vi "C400_module.vi"() -> ()   [LabVIEW 2018]
uses:
  data/resilio/Dropbox/rnd/LabView/2p_scanners/notifiers/EventNames.ctl
  data/resilio/Dropbox/rnd/LabView/2p_scanners/notifiers/notifierMessages.ctl
panel:
  in  "autoconnect":bool=TRUE
  out "Ch1 Position Units":string
  out "Ch1Range":i32
  in  "Read Sensor":bool
  out "Ch1 Sensor Value":dbl format="%.3f"
  out "Serial Numbers":string[](array[string])
  out "FT_Status":u64(ring) items=["FT_OK", "FT_INVALID_HANDLE", "FT_DEVICE_NOT_FOUND", "FT_DEVICE_NOT_OPENED", "FT_IO_ERROR", "FT_INSUFFICIENT_RESOURCES", "FT_INVALID_PARAMETER", "FT_INVALID_BAUD_RATE", "FT_DEVICE_NOT_OPENED_FOR_ERASE", "FT_DEVICE_NOT_OPENED_FOR_WRITE", "FT_FAILED_TO_WRITE_DEVICE", "FT_EEPROM_READ_FAILED", "FT_EEPROM_WRITE_FAILED", "FT_EEPROM_ERASE_FAILED", "FT_EEPROM_NOT_PRESENT", "FT_EEPROM_NOT_PROGRAMMED", "FT_INVALID_ARGS", "FT_NOT_SUPPORTED", "FT_OTHER_ERROR"]
  in  "Ch1 Position Cmd":dbl format="%.3f"
  in  "Connect":bool
  in  "Stop VI":bool caption="Stop Button"
  in  "Listbox":i32(listbox)=-1
  in  "Handle":u64
  # "FT_Status displays the error type if an\nFTDI USB function did not execute properly."
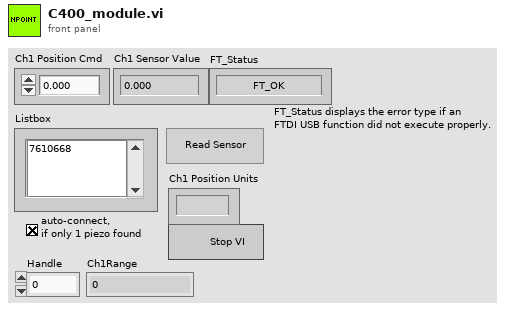
[diagram p1: front panel]
types:
  T1 = typedef "notifierMessages.ctl" = cluster{"data":variant, "source":string, "time tick":u32}
  T2 = typedef "EventNames.ctl" = enum16{"None", "rig shutter", "expStarted", "frameAcq", "stim", "zStage", "DAQ/galvo", "piezo", "liqLens", "expEnded"}
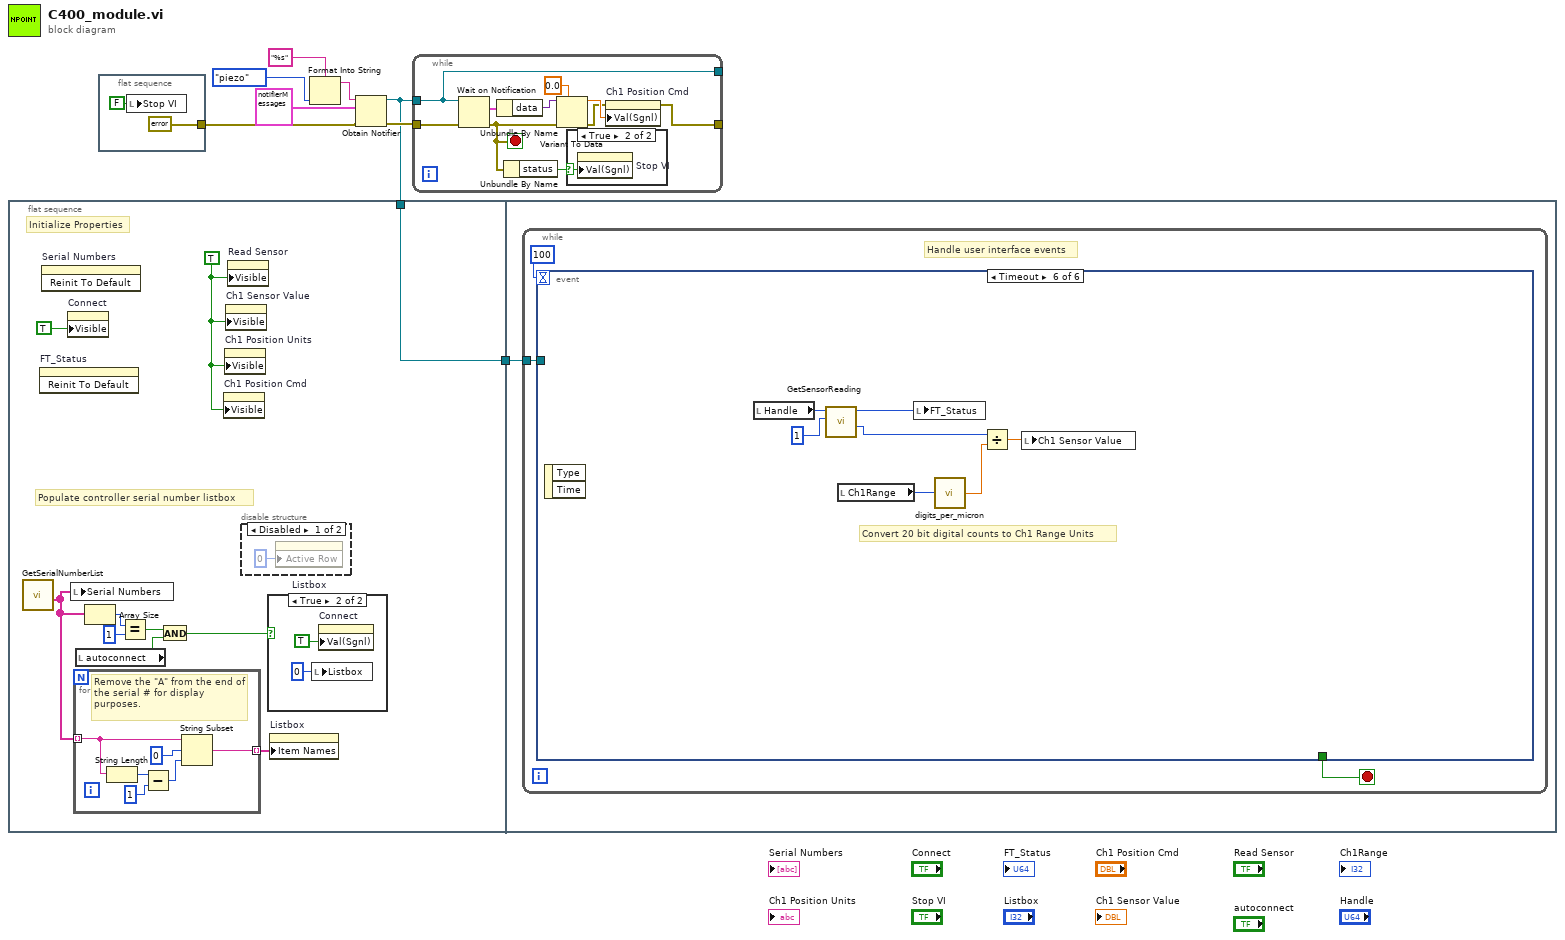
[diagram p0: block diagram]
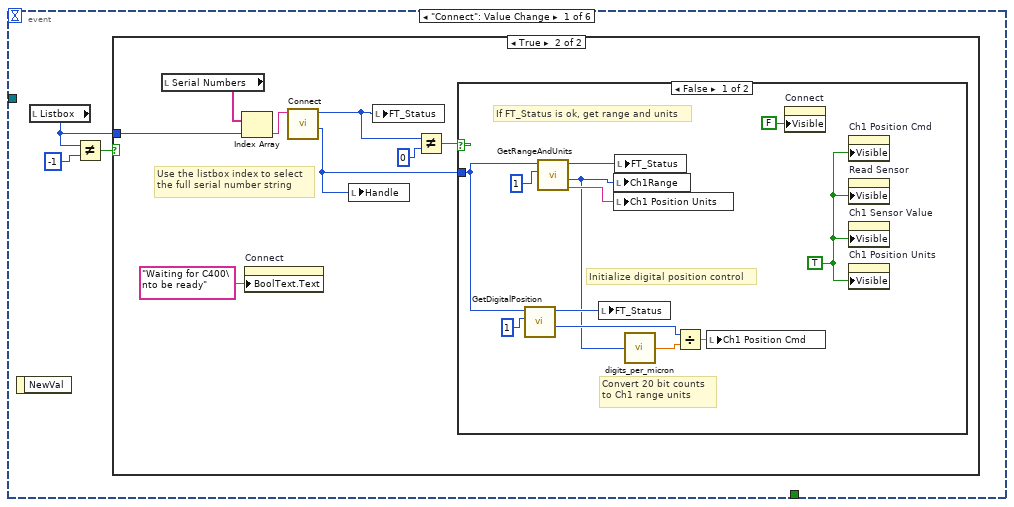
[diagram p5: hidden frame]
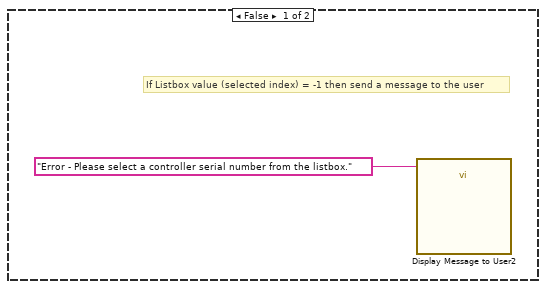
[diagram p6: hidden frame]
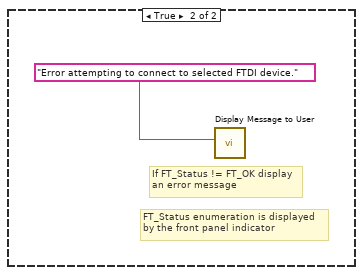
[diagram p7: hidden frame]
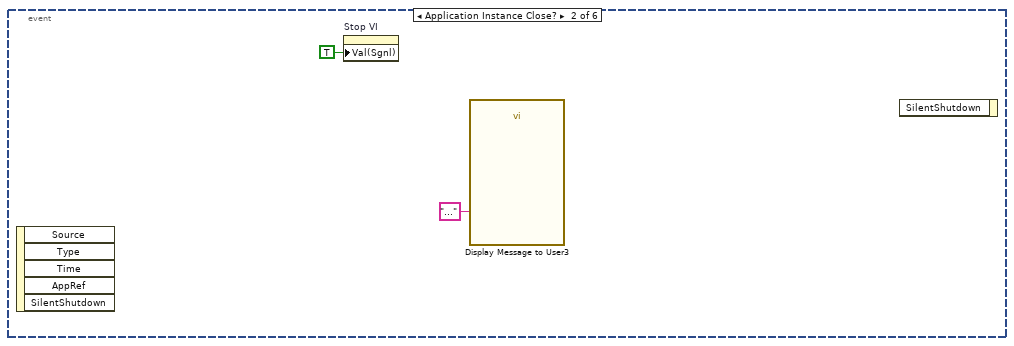
[diagram p8: hidden frame]
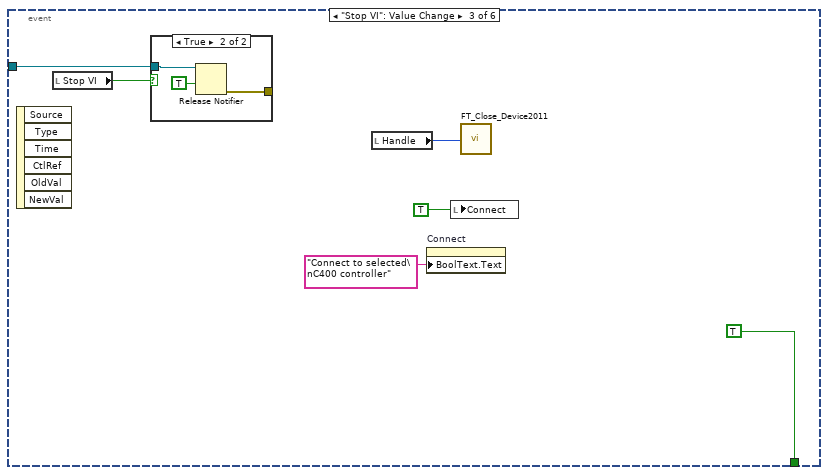
[diagram p9: hidden frame]
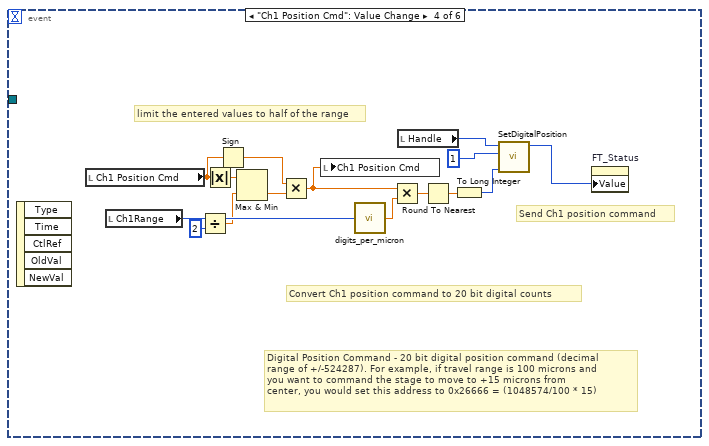
[diagram p11: hidden frame]
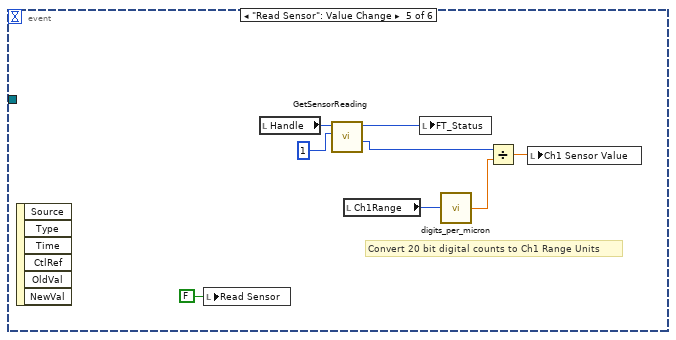
[diagram p12: hidden frame]
diagram:
  n1 = flat-sequence {
    tunnel: w2 -> [w9]
    tunnel: [w9] -> w1
    tunnel: w1 -> [w28]
    frame #0 {
      w16 = TRUE ("Visible")
      # "Initialize Properties"
      # "Populate controller serial number listbox"
      n2 = call "GetSerialNumberList.vi"() -> ("C400 Serial Number Array"=w10:string[])  [unwired: 11 in]
      n3 = invoke on="FT_Status" class="Ring (strict)" method="Reinit To Default"() -> ()  [unwired: 3 in, 3 out]
      n4 = invoke on="Serial Numbers" class="Arr (strict)" method="Reinit To Default"() -> ()  [unwired: 3 in, 3 out]
      n5 = property on="Connect" class="Bool (strict)"("Visible"=TRUE) -> ()  [unwired: 2 in, 2 out]
      n6 = local write "Serial Numbers"(w10) -> ()
      n7 = for {
        tunnel: [w23] -> w18 mode=indexing
        tunnel: w10 -> [w22] mode=indexing
        # "Remove the \"A\" from the end of the serial # for display purposes."
        n8 = String Length(string=w22) -> (length=w26:i32)
        n9 = Subtract(x=w26, y=1) -> (x-y=w24:i32)
        n10 = String Subset(string=w22, offset (0)=0, length (rest)=w24) -> (substring=w23:string)
      }
      n11 = local read "autoconnect"() -> (w12:bool)
      n12 = Array Size(array=w10) -> (size(s)=w14:i32)
      n13 = Equal?(x=w14, y=1) -> (x = y?=w11:bool)
      n14 = And(x=w11, y=w12) -> (x .and. y?=w15:bool)
      n15 = property on="Ch1 Position Cmd" class="DigNum (strict)"("Visible"=w16) -> ()  [unwired: 2 in, 2 out]
      n16 = property on="Ch1 Position Units" class="Str"("Visible"=w16) -> ()  [unwired: 2 in, 2 out]
      n17 = property on="Ch1 Sensor Value" class="DigNum (strict)"("Visible"=w16) -> ()  [unwired: 2 in, 2 out]
      n18 = property on="Read Sensor" class="Bool (strict)"("Visible"=w16) -> ()  [unwired: 2 in, 2 out]
      n19 = disable-structure shown="Disabled" {
        frame Disabled {
          n20 = property on="Listbox" class="LstBox (strict)"("Active Row"=0 ("Active Row:Active Row Number")) -> ()  [unwired: 2 in, 2 out]
        }
        frame Enabled {
        }
      }
      n21 = case shown="True" w15 {
        frame False {
        }
        frame True {
          n22 = local write "Listbox"(0 ("Listbox")) -> ()
          n23 = property on="Connect" class="Bool (strict)"("Val(Sgnl)"=TRUE ("Value (Signaling)")) -> ()  [unwired: 2 in, 2 out]
        }
      }
      n24 = property on="Listbox" class="LstBox (strict)"("Item Names"=w18) -> ()  [unwired: 2 in, 2 out]
    }
    frame #1 {
      n25 = while {
        tunnel: w28 -> [w29]
        stop <- w31 stop-if-true
        # "Handle user interface events"
        n26 = event shown="[5] Timeout" {
          selector: _ -> [_ _ _ _ _ _]
          dyn-events: _ -> [_ _ _ _ _ _]
          timeout: 100 -> [_ _ _ _ _ _]
          tunnel: [_ _ TRUE _ _ _] -> w31
          tunnel: w29 -> [_ _ w59 _ _ _]
          event "Connect": Value Change {
            n27 = event-data() -> ()  [unwired: 1 in, 1 out]
            n28 = local read "Listbox"() -> (w32:i32)
            n29 = Not Equal?(x=w32, y=-1) -> (x != y?=w34:bool)
            n30 = case shown="True" w34 {
              tunnel: w32 -> [_ w43]
              frame False {
                # "If Listbox value (selected index) = -1 then send a message to the user"
                n31 = call "Display Message to User2"("Message"="Error - Please select a controller serial number from the listbox.") -> ()  [unwired: 9 in, 2 out]
              }
              frame True {
                # "Use the listbox index to select\nthe full serial number string"
                n32 = local read "Serial Numbers"() -> (w38:string[])
                n33 = Index Array(array=w38, index=w43) -> (element=w39:string)
                n34 = property on="Connect" class="Bool (strict)"("BoolText.Text"="Waiting for C400\nto be ready" ("Boolean Text.Text")) -> ()  [unwired: 2 in, 2 out]
                n35 = call "Connect.vi"("Device Serial Number"=w39) -> ("Handle"=w42:u64, "FT_Status"=w37:u64)  [unwired: 9 in]
                n36 = local write "Handle"(w42) -> ()
                n37 = local write "FT_Status"(w37) -> ()
                n38 = Not Equal?(x=w37, y=u64 0) -> (x != y?=w40:bool)
                n39 = case shown="False" w40 {
                  tunnel: w42 -> [w49 _]
                  frame False {
                    w46 = TRUE ("Visible")
                    # "Convert 20 bit counts\nto Ch1 range units"
                    # "Initialize digital position control"
                    # "If FT_Status is ok, get range and units"
                    n40 = call "GetDigitalPosition.vi"("Handle"=w49, "Controller Channel"=i64 1) -> ("FT_Status"=w47:u64, "Position"=w53:i64)  [unwired: 7 in]
                    n41 = call "GetRangeAndUnits.vi"("Handle"=w49, "Controller Channel"=i64 1) -> ("FT_Status"=w51:u64, "Range"=w44:i32, "Range Units"=w50:string)  [unwired: 6 in]
                    n42 = local write "FT_Status"(w47) -> ()
                    n43 = local write "Ch1Range"(w44) -> ()
                    n44 = local write "Ch1 Position Units"(w50) -> ()
                    n45 = local write "FT_Status"(w51) -> ()
                    n46 = call "digits_per_micron.vi"("Ch1Range"=w44) -> ("digital_per_micron"=w45:dbl)
                    n47 = Divide(x=w53, y=w45) -> (x/y=w48:dbl)
                    n48 = local write "Ch1 Position Cmd"(w48) -> ()
                    n49 = property on="Connect" class="Bool (strict)"("Visible"=FALSE) -> ()  [unwired: 2 in, 2 out]
                    n50 = property on="Ch1 Position Cmd" class="DigNum (strict)"("Visible"=w46) -> ()  [unwired: 2 in, 2 out]
                    n51 = property on="Read Sensor" class="Bool (strict)"("Visible"=w46) -> ()  [unwired: 2 in, 2 out]
                    n52 = property on="Ch1 Sensor Value" class="DigNum (strict)"("Visible"=w46) -> ()  [unwired: 2 in, 2 out]
                    n53 = property on="Ch1 Position Units" class="Str"("Visible"=w46) -> ()  [unwired: 2 in, 2 out]
                  }
                  frame True {
                    # "FT_Status enumeration is displayed\nby the front panel indicator"
                    # "If FT_Status != FT_OK display\nan error message"
                    n54 = call "Display Message to User"("Message"="Error attempting to connect to selected FTDI device.") -> ()  [unwired: 9 in, 2 out]
                  }
                }
              }
            }
          }
          event Application Instance Close? {
            n55 = event-data() -> ()  [unwired: 1 in, 5 out]
            n56 = property on="Stop VI" class="Bool (strict)"("Val(Sgnl)"=TRUE ("Value (Signaling)")) -> ()  [unwired: 2 in, 2 out]
            n57 = call "Display Message to User3"("Message"="...") -> ()  [unwired: 9 in, 2 out]
            n58 = event-data() -> ()  [unwired: 2 in, 1 out]
          }
          event "Stop VI": Value Change {
            n59 = event-data() -> ()  [unwired: 1 in, 6 out]
            n60 = local read "Stop VI"() -> (w60:bool)
            n61 = case shown="True" w60 {
              tunnel: [_ w66] -> _
              tunnel: w59 -> [_ w65]
              frame False {
              }
              frame True {
                n62 = Release Notifier(notifier=w65, force destroy? (F)=TRUE) -> (error out=w66:errorcluster)  [unwired: 1 in, 2 out]
              }
            }
            n63 = local read "Handle"() -> (w62:u64)
            n64 = property on="Connect" class="Bool (strict)"("BoolText.Text"="Connect to selected\nC400 controller" ("Boolean Text.Text")) -> ()  [unwired: 2 in, 2 out]
            n65 = local write "Connect"(TRUE ("Visible")) -> ()
            n66 = call "FT_Close_Device2011.vi"("Handle"=w62) -> ()  [unwired: 1 out]
          }
          event "Ch1 Position Cmd": Value Change {
            # "limit the entered values to half of the range"
            # "Digital Position Command - 20 bit digital position command (decimal\nrange of +/-524287). For example, if travel range is 100 microns and\nyou want to command the stage to move to +15 microns from\ncenter, you would set this address to 0x26666 = (1048574/100 * 15)"
            # "Send Ch1 position command"
            # "Convert Ch1 position command to 20 bit digital counts"
            n67 = event-data() -> ()  [unwired: 1 in, 5 out]
            n68 = local read "Ch1 Position Cmd"() -> (w71:dbl)
            n69 = local read "Ch1Range"() -> (w75:i32)
            n70 = Divide(x=w75, y=2) -> (x/y=w73:dbl)
            n71 = Absolute Value(x=w71) -> (abs(x)=w72:dbl)
            n72 = Sign(1:w71) -> (0:w69:dbl)
            n73 = Max & Min(x=w72, y=w73) -> (min(x,y)=w70:dbl)  [unwired: 1 out]
            n74 = Multiply(x=w69, y=w70) -> (x*y=w68:dbl)
            n75 = local write "Ch1 Position Cmd"(w68) -> ()
            n76 = call "digits_per_micron.vi"("Ch1Range"=w75) -> ("digital_per_micron"=w76:dbl)
            n77 = Multiply(x=w68, y=w76) -> (x*y=w80:dbl)
            n78 = local read "Handle"() -> (w77:u64)
            n79 = Round To Nearest(number=w80) -> (nearest integer value=w79:dbl)
            n80 = To Long Integer(number=w79) -> (32bit integer=w78:i32)
            n81 = call "SetDigitalPosition.vi"("Position"=w78, "Controller Channel"=i64 1, "Handle"=w77) -> ("FT_Status"=w81:u64)  [unwired: 8 in]
            n82 = property on="FT_Status" class="Ring (strict)"("Value"=w81) -> ()  [unwired: 2 in, 2 out]
          }
          event "Read Sensor": Value Change {
            # "Convert 20 bit digital counts to Ch1 Range Units"
            n83 = event-data() -> ()  [unwired: 1 in, 6 out]
            n84 = local write "Read Sensor"(FALSE ("Read Sensor")) -> ()
            n85 = local read "Handle"() -> (w87:u64)
            n86 = call "GetSensorReading.vi"("Handle"=w87, "Controller Channel"=i64 1) -> ("FT_Status"=w88:u64, "Sensor Reading"=w89:i64)  [unwired: 7 in]
            n87 = local read "Ch1Range"() -> (w84:i32)
            n88 = local write "FT_Status"(w88) -> ()
            n89 = call "digits_per_micron.vi"("Ch1Range"=w84) -> ("digital_per_micron"=w85:dbl)
            n90 = Divide(x=w89, y=w85) -> (x/y=w86:dbl)
            n91 = local write "Ch1 Sensor Value"(w86) -> ()
          }
          event Timeout {
            # "Convert 20 bit digital counts to Ch1 Range Units"
            n92 = event-data() -> ()  [unwired: 1 in, 2 out]
            n93 = local read "Handle"() -> (w95:u64)
            n94 = call "GetSensorReading.vi"("Handle"=w95, "Controller Channel"=i64 1) -> ("FT_Status"=w96:u64, "Sensor Reading"=w97:i64)  [unwired: 7 in]
            n95 = local read "Ch1Range"() -> (w92:i32)
            n96 = local write "FT_Status"(w96) -> ()
            n97 = call "digits_per_micron.vi"("Ch1Range"=w92) -> ("digital_per_micron"=w93:dbl)
            n98 = Divide(x=w97, y=w93) -> (x/y=w94:dbl)
            n99 = local write "Ch1 Sensor Value"(w94) -> ()
          }
        }
      }
    }
  }
  n100 = flat-sequence {
    tunnel: [errorcluster {"status"=FALSE, "code"=0, "source"=""} ("error in (no error)")] -> w4
    frame #0 {
      n101 = local write "Stop VI"(FALSE ("stop")) -> ()
    }
  }
  n102 = Format Into String(format string="%s", EventNames."piezo" ("NotifierName")) -> (resulting string=w6:string)  [unwired: 2 in, 1 out]
  n103 = Obtain Notifier(name (unnamed)=w6, notification data type=T1 {"data"=variant, "source"="", "time tick"=0} ("mess"), error in (no error)=w4) -> (notifier out=w2:refnum<notifier>, error out=w3:errorcluster)  [unwired: 1 in, 1 out]
  n104 = while {
    tunnel: w2 -> [w102]
    tunnel: w3 -> [w109]
    tunnel: [w103] -> _
    tunnel: [w102] -> _
    stop <- w101 stop-if-true
    n105 = Wait on Notification(notifier=w102, error in (no error)=w109) -> (notification=w108:T1, error out=w101:errorcluster)  [unwired: 2 in, 2 out]
    n106 = Unbundle By Name(w108) -> ("data"=w107:variant)
    n107 = Unbundle By Name(w101) -> ("status"=w100:bool)
    n108 = Variant To Data(error in=w101, type=0.0, Variant=w107) -> (data=w105:dbl, error out=w104:errorcluster)
    n109 = case shown="True" w100 {
      selector: w100 -> [_ w110]
      frame False {
      }
      frame True {
        n110 = property on="Stop VI" class="Bool (strict)"("Val(Sgnl)"=w110) -> ()  [unwired: 2 in, 2 out]
      }
    }
    n111 = property on="Ch1 Position Cmd" class="DigNum (strict)"(error in=w104, "Val(Sgnl)"=w105) -> (error out=w103:errorcluster)  [unwired: 1 in, 1 out]
  }
